vi "init.vi"(0 "EXC2Test in":refnum<class "EXC2Test.lvclass">, 1 "Tolerance":dbl[unit], 5 "Log":refnum<class "ITestLog.lvclass">, 7 "DAQ Channel To Read":refnum<k21>, 9 "Expected Value":dbl[unit], 11 "error in (no error)":errorcluster, 12 "Samples To Read":dbl) -> (4 "EXC2Test out":refnum<class "EXC2Test.lvclass">, 15 "error out":errorcluster)   [LabVIEW 2015, in "EXC2Test.lvclass"]
uses:
  EXC2Test.lvclass
  Model/TestLog/ITestLog/ITestLog.lvclass
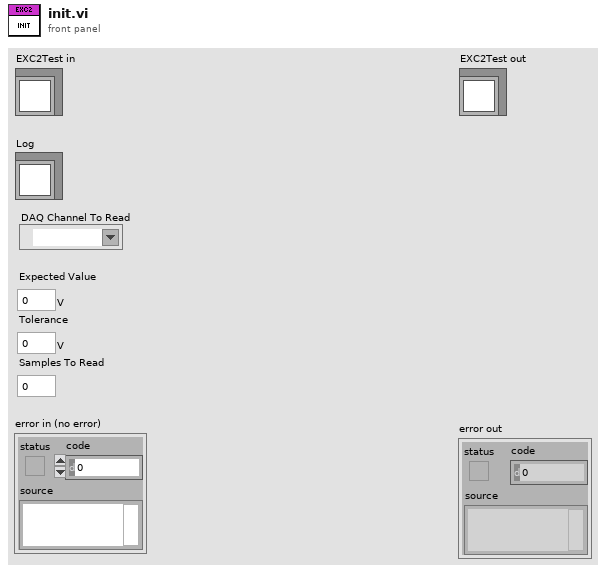
[diagram p1: front panel]
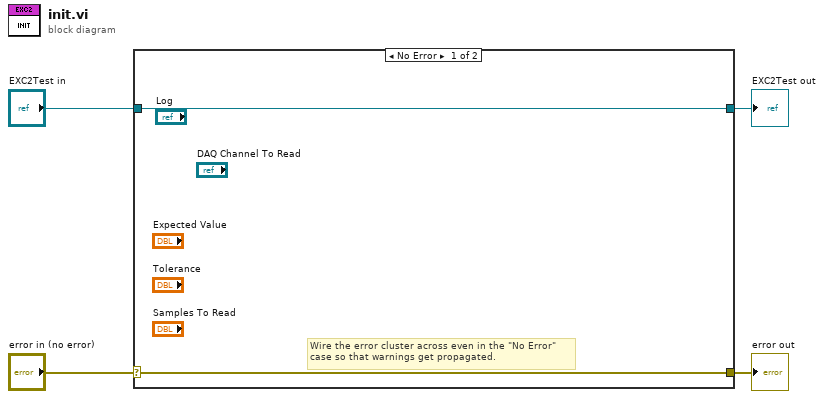
[diagram p0: block diagram]
diagram:
  n1 = case shown="No Error" "error in (no error)" {
    selector: "error in (no error)" -> [w5 w8]
    tunnel: [w5 w8] -> w3
    tunnel: [w6 w7] -> w1
    tunnel: "EXC2Test in" -> [w6 w7]
    frame No Error {
      # "Wire the error cluster across even in the \"No Error\"\ncase so that warnings get propagated."
    }
    frame Error {
    }
  }
  "error out" <- w3
  "EXC2Test out" <- w1
